vi "Read.vi"(11 "ApiArrayValue in":refnum<class "ApiArrayValue.lvclass">) -> (2 "APIs":refnum<class "API.lvclass">[](array[class]))   [LabVIEW 2020, in "Volatus.lvlib" / "ApiArrayValue.lvclass"]
uses:
  ApiArrayValue.lvclass
  ApiArrayValue.lvclass/ApiArrayValue.ctl
  API/API.lvclass
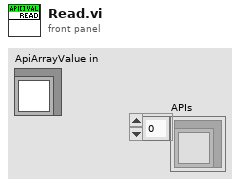
[diagram p1: front panel]
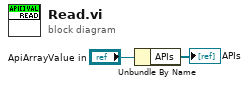
[diagram p0: block diagram]
diagram:
  n1 = Unbundle By Name("ApiArrayValue in") -> ("APIs"=→"APIs":refnum<class "API.lvclass">[])
